vi "LCD_Simulaation.vi"(8 "error in (no error)":errorcluster, 11 "Refnum in":T1) -> (0 "error out":errorcluster, 3 "Refnum out":T1)   [LabVIEW 2019]
uses:
  <vilib>/vision/Image Controls.llb/IMAQ Image.ctl
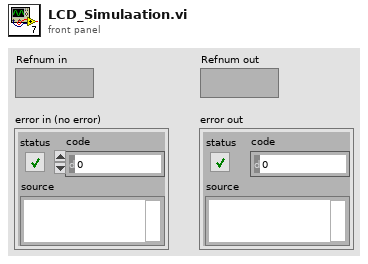
[diagram p1: front panel]
types:
  T1 = typedef "IMAQ Image.ctl" = refnum<image>
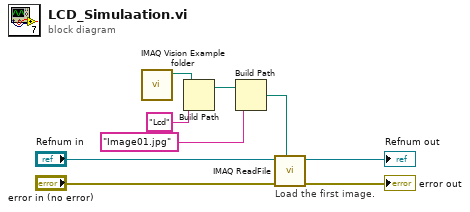
[diagram p0: block diagram]
diagram:
  # "Load the first image."
  n1 = call "IMAQ Vision Example folder.vi"() -> ("Example Image Path"=w5:path)  [unwired: 11 in]
  n2 = Build Path(base path=w5, name or relative path="Lcd") -> (appended path=w4:path)
  n3 = Build Path(base path=w4, name or relative path="Image01.jpg") -> (appended path=w6:path)
  n4 = call "IMAQ ReadFile"("File Path"=w6, "error in (no error)"="error in (no error)", "Image"="Refnum in") -> ("error out"=→"error out":errorcluster, "Image Out"=→"Refnum out":T1)  [unwired: 2 in, 5 out]
